vi "Intake Shooter Controller.vi"(8 "error in":errorcluster) -> ()   [LabVIEW 2019]
doc: "This VI executes continuously carrying out the current operation and responding to updates or new operations. It will often contain the timing or control code that is difficult to place directly in TeleOp. This VI generally opens all sensors and motors and isolates the rest of the robot code from knowing how the operations are carried out."
uses:
  <vilib>/Rock Robotics/WPI/Framework/Completion Status.ctl
  Intake Shooter Setpoints.ctl
  Intake Shooter Operations.ctl
  <vilib>/Rock Robotics/WPI/ThirdParty/REV Robotics/SPARK MAX/Typedef/Spark MAX Idle Mode.ctl
  <vilib>/Rock Robotics/WPI/ThirdParty/REV Robotics/SPARK MAX/Typedef/Spark MAX Control Type.ctl
  <vilib>/Rock Robotics/WPI/ThirdParty/Phoenix-LabVIEW/Motor Controller/Controls/CTRE_Phoenix_MotorControl_ControlMode.ctl
  <vilib>/Rock Robotics/Network Tables/NT Write Boolean.vi
panel:
  out "Iterations 3":i32
  out "Analog Position 2":dbl
  out "Iterations 2":i32
  out "Iterations":i32
  out "Analog Position":dbl
  in  "Interactive Values":T1
  out "Current\nCmd":string
  in  "Buttons":cluster{"Execute Cmd":bool, "Abort Cmd":bool}
  out "Command Timing":cluster{"Start Time (ms)":u32, "Iterations":i32}
  out "Status":T3
  # "Tip: It may be helpful to observe inputs and sensor values.\nYou may also want to display tuning or debugging controls."
  # "Interactive Command: You may fill in the settings for a command\nand schedule it with the Execute button. You can observe and abort\nany command while fine tuning the code for the controller."
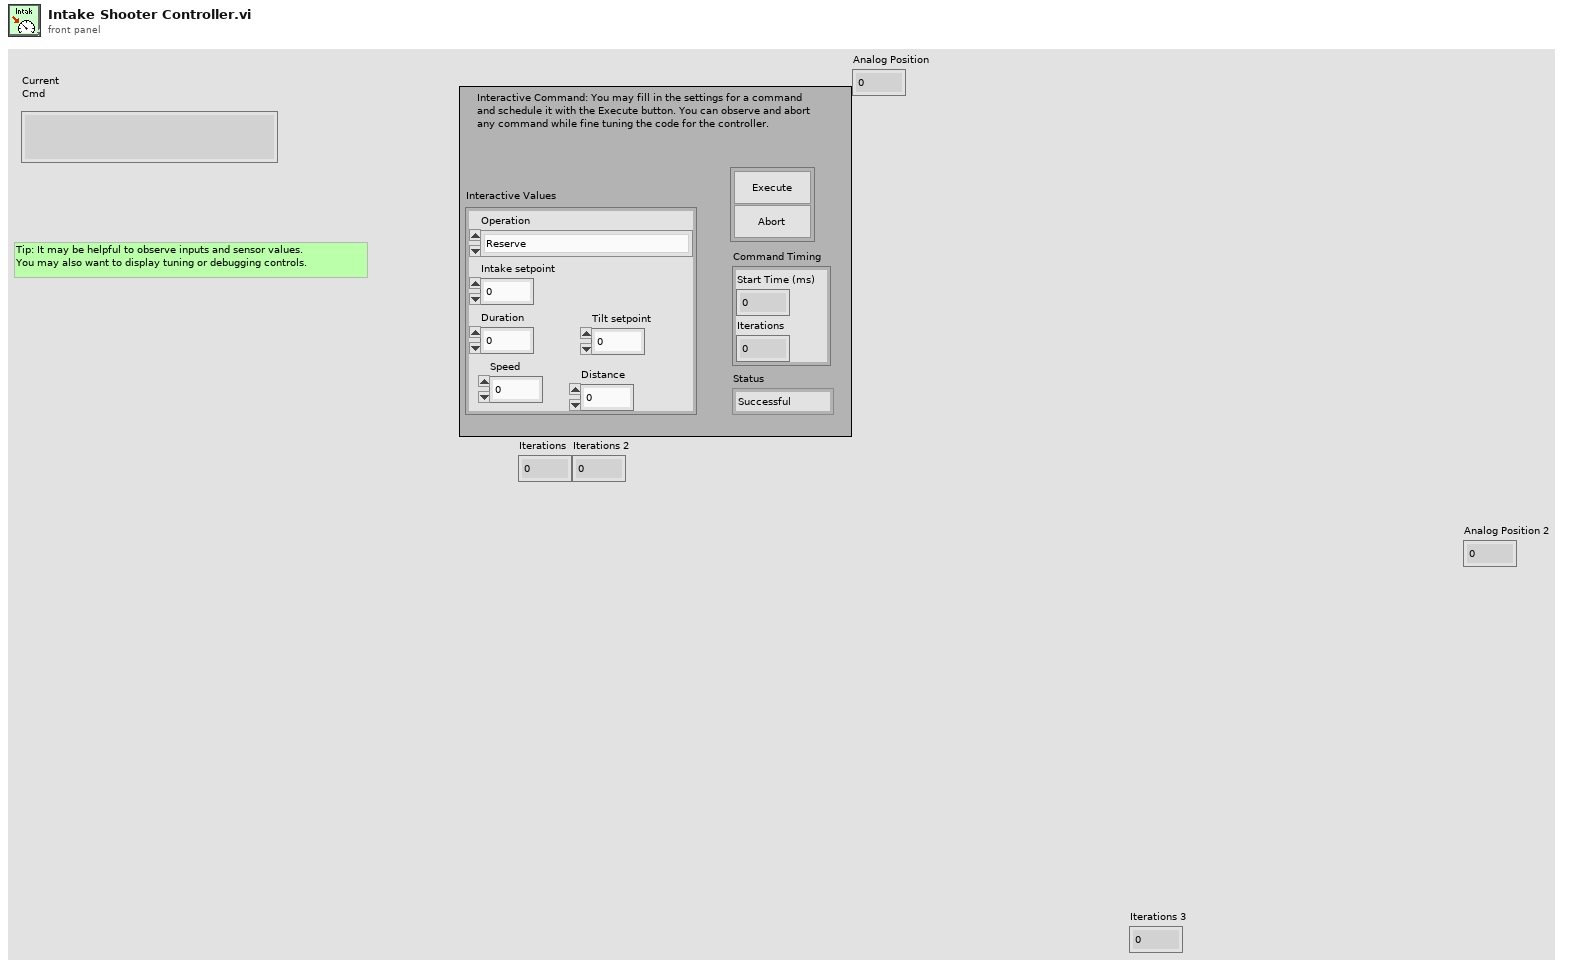
[diagram p1: front panel]
types:
  T1 = typedef "Intake Shooter Setpoints.ctl" = cluster{"Operation":T2, "Intake setpoint":dbl, "Duration":dbl, "Tilt setpoint":dbl, "Speed":dbl, "Distance":dbl}
  T2 = typedef "Intake Shooter Operations.ctl" = enum16{"Reserve", "Read Current", "Immediate", "Go up", "Go down", "Armediate"}
  T3 = typedef "Completion Status.ctl" = enum16{"Successful", "Aborted", "Incomplete"}
  T4 = typedef "Spark MAX Idle Mode.ctl" = enum16{"Coast", "Brake"}
  T5 = typedef "WPI_MotorControlDeviceRef.ctl" = cluster{"DeviceStatus":errorcluster, "Type":T6, "PWM":cluster{"PWM Channel":T7, "DeadBand":T8}, "CAN":cluster{"Device Number":u8, "SetOutput VI Ref":variant, "GetOutput VI Ref":variant, "Enable VI Ref":variant, "Disable VI Ref":variant, "Data":variant}, "Invert":bool, "DIO PWM":cluster{"PWM \"Enable\" Channel":T7, "DIOChannel":T9, "PWM Rate":dbl}}
  T6 = typedef "WPI_MotorControlType.ctl" = enum16{"PWM", "CAN", "DIO PWM"}
  T7 = typedef "FPGA_DIOPWMChannel.ctl" = enum8{"PWM 0", "PWM 1", "PWM 2", "PWM 3", "PWM 4", "PWM 5", "PWM 6", "PWM 7", "PWM 8", "PWM 9", "PWM MXP 0", "PWM MXP 1", "PWM MXP 2", "PWM MXP 3", "PWM MXP 4", "PWM MXP 5", "PWM MXP 6", "PWM MXP 7", "PWM MXP 8", "PWM MXP 9", "Invalid"}
  T8 = typedef "WPI_PWMDeadband.ctl" = cluster{"Name":string, "maxPositivePwm":i32, "minPositivePwm":i32, "centerPwm":i32, "maxNegativePwm":i32, "minNegativePwm":i32, "angularRange":u16}
  T9 = typedef "FPGA_DIOChannel.ctl" = enum8{"DIO 0", "DIO 1", "DIO 2", "DIO 3", "DIO 4", "DIO 5", "DIO 6", "DIO 7", "DIO 8", "DIO 9", "DIO MXP 0", "DIO MXP 1", "DIO MXP 2", "DIO MXP 3", "DIO MXP 4", "DIO MXP 5", "DIO MXP 6", "DIO MXP 7", "DIO MXP 8", "DIO MXP 9", "DIO MXP 10", "DIO MXP 11", "DIO MXP 12", "DIO MXP 13", "DIO MXP 14", "DIO MXP 15", "SPI Port CS1", "SPI Port CS2", "SPI Port CS3", "SPI Port MISO", "SPI Port MOSI", "Invalid"}
  T10 = typedef "Command Status Info.ctl" = cluster{"Name":string, "Status":T3, "notifier out":T11}
  T11 = typedef "Completion Notifier.ctl" = refnum<notifier>
  T12 = cluster{"Current Command":T1, "Command Timing":cluster{"Start Time (ms)":u32, "Iterations":i32}, "Command Arguments":cluster{"Command Info":T10, "Description":string, "Default Command":T1, "queue out":refnum<queue>, "Subsystem Name":string}}
  T13 = typedef "Spark MAX Control Type.ctl" = enum16{"Percent VBus", "Voltage", "Velocity", "Position", "Smart Motion", "Current", "Smart Velocity"}
  T14 = typedef "CTRE_Phoenix_MotorControl_ControlMode.ctl" = u16
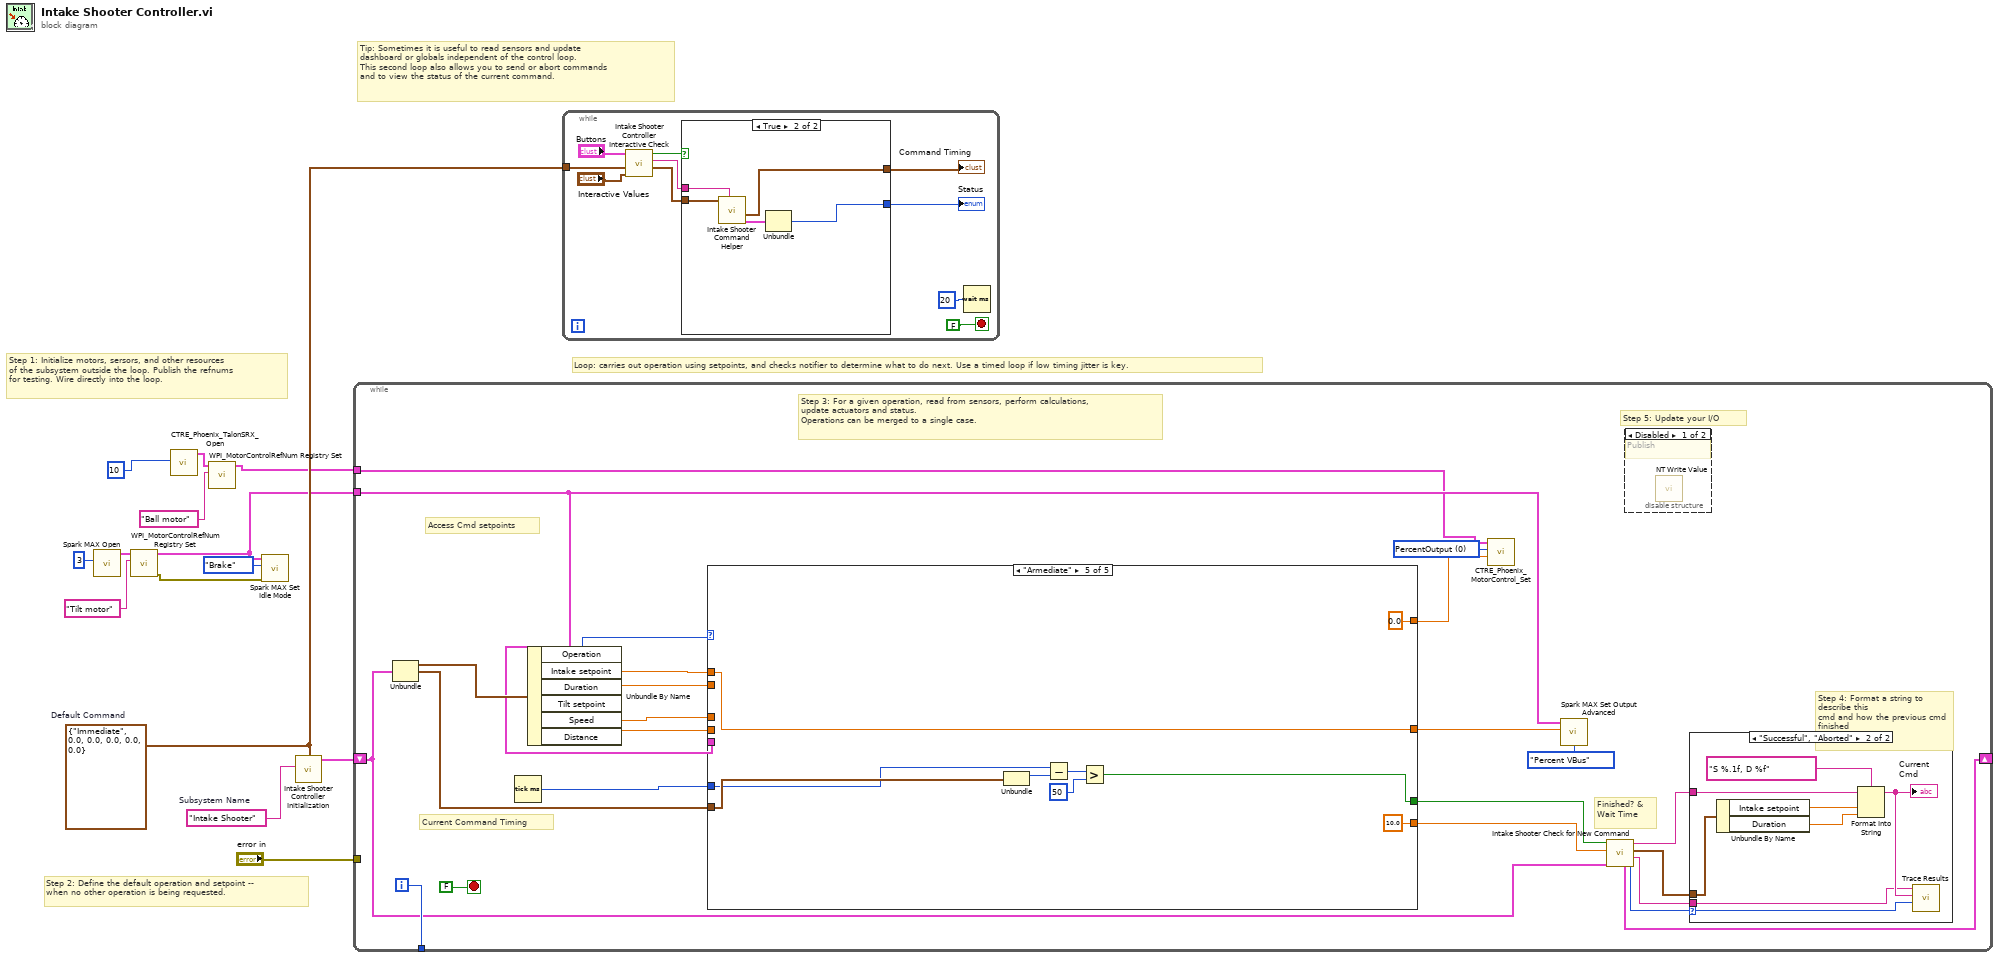
[diagram p0: block diagram]
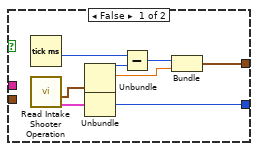
[diagram p2: hidden frame]
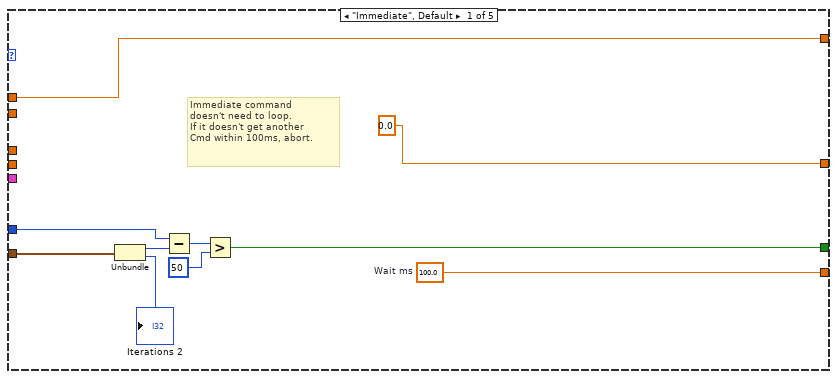
[diagram p4: hidden frame]
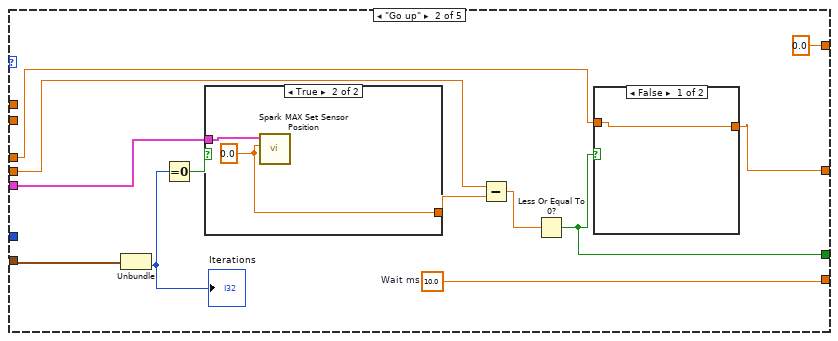
[diagram p5: hidden frame]
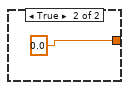
[diagram p6: hidden frame]
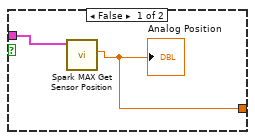
[diagram p7: hidden frame]
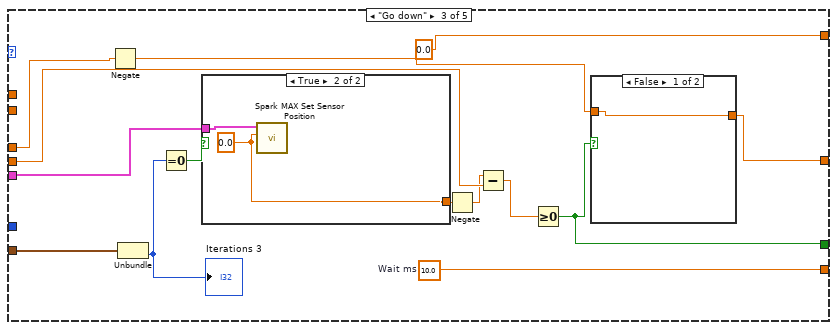
[diagram p8: hidden frame]
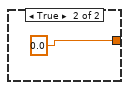
[diagram p9: hidden frame]
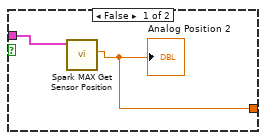
[diagram p10: hidden frame]
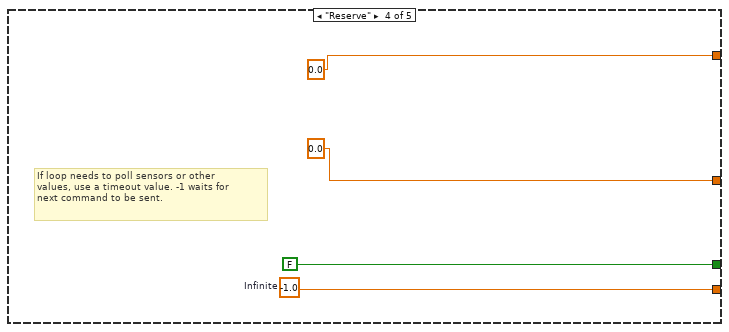
[diagram p11: hidden frame]
diagram:
  w11 = T1 {"Operation"=enum."Immediate", "Intake setpoint"=0.0, "Duration"=0.0, "Tilt setpoint"=0.0, "Speed"=0.0, "Distance"=0.0}  # Default Command
  w12 = "Intake Shooter"  # Subsystem Name
  # "Tip: Sometimes it is useful to read sensors and update\ndashboard or globals independent of the control loop.\nThis second loop also allows you to send or abort commands\nand to view the status of the current command."
  # "Step 2: Define the default operation and setpoint --\nwhen no other operation is being requested."
  # "Step 1: Initialize motors, sersors, and other resources\nof the subsystem outside the loop. Publish the refnums\nfor testing. Wire directly into the loop."
  # "Loop: carries out operation using setpoints, and checks notifier to determine what to do next. Use a timed loop if low timing jitter is key."
  n1 = call <vilib>:"Spark MAX Open.vi"("Device Number"=u8 3) -> ("MotorControlDeviceRef"=w9:T5)  [unwired: 9 in, 1 out]
  n2 = call <vilib>:"WPI_MotorControlRefNum Registry Set.vi"("refnum name"="Tilt motor", "MotorControlDevRef"=w9) -> ("error out"=w3:errorcluster, "MotorControlDevRef"=w2:T5)  [unwired: 8 in]
  n3 = call <vilib>:"CTRE_Phoenix_TalonSRX_Open.vi"("Device Number"=u8 10) -> ("CAN Talon SRX Ref"=w4:T5)  [unwired: 9 in, 1 out]
  n4 = call <vilib>:"WPI_MotorControlRefNum Registry Set.vi"("refnum name"="Ball motor", "MotorControlDevRef"=w4) -> ("MotorControlDevRef"=w6:T5)  [unwired: 8 in, 1 out]
  n5 = call <vilib>:"Spark MAX Set Idle Mode.vi"("error in (no error)"=w3, "Idle Mode"=Spark_MAX_Idle_Mode."Brake", "MotorControlDeviceRef in"=w2) -> ()  [unwired: 7 in, 2 out]
  n6 = call "Intake Shooter Controller Initialization.vi"("Subsystem Name"=w12, "Default Command"=w11) -> ("Current Command"=w13:T12)  [unwired: 9 in]
  n7 = while {
    shift-right: [w31] -> _
    shift-left: w13 -> [w24]
    tunnel: [w37] -> _
    tunnel: "error in" -> [_]
    tunnel: w6 -> [w17]
    tunnel: w2 -> [w19]
    i -> [w37]
    stop <- FALSE stop-if-true
    w15 = T14 0 items=["PercentOutput"=0, "Position"=1, "Velocity"=2, "Current"=3, "Follower"=5, "MotionProfile"=6, "MotionMagic"=7, "MotionProfileArc"=10, "Disabled"=15] ("Control Mode")
    # "Step 5: Update your I/O"
    # "Step 4: Format a string to describe this\ncmd and how the previous cmd finished"
    # "Current Command Timing"
    # "Access Cmd setpoints"
    # "Finished? &\nWait Time"
    # "Step 3: For a given operation, read from sensors, perform calculations,\nupdate actuators and status.\nOperations can be merged to a single case."
    n8 = Unbundle(w24) -> ("Current Command"=w36:T1, "Command Timing"=w33:cluster{"Start Time (ms)":u32, "Iterations":i32})  [unwired: 1 out]
    n9 = Tick Count (ms)() -> (millisecond timer value=w34:u32)
    n10 = Unbundle By Name(w36) -> ("Operation"=w35:T2, "Intake setpoint"=w32:dbl, "Duration"=w22:dbl, "Speed"=w21:dbl, "Distance"=w20:dbl)  [unwired: 1 out]
    n11 = case shown="\"Armediate\"" w35 {
      tunnel: [w48 w60 w71 w90 10.0 ("Infinite")] -> w29
      tunnel: [w42 w50 w72 FALSE ("ignore previous (F)") w93] -> w30
      tunnel: w33 -> [w44 w59 w70 _ w94]
      tunnel: w34 -> [w43 _ _ _ w92]
      tunnel: w32 -> [w41 _ _ _ w98]
      tunnel: [w41 0.0 ("f") 0.0 ("f") 0.0 ("f") 0.0 ("f")] -> w16
      tunnel: [0.0 ("Setpoint") w52 w73 0.0 w98] -> w23
      tunnel: w19 -> [_ w56 w76 _ _]
      tunnel: w22 -> [_ _ _ _ _]
      tunnel: w21 -> [_ w51 w75 _ _]
      tunnel: w20 -> [_ w55 w69 _ _]
      frame "Immediate", Default {
        w48 = 100.0  # Wait ms
        # "Immediate command\ndoesn't need to loop.\nIf it doesn't get another\nCmd within 100ms, abort."
        n12 = Unbundle(w44) -> ("Start Time (ms)"=w47:u32, "Iterations"=→"Iterations 2":i32)
        n13 = Subtract(x=w43, y=w47) -> (x-y=w46:u32)
        n14 = Greater?(x=w46, y=u8 50 ("Left Motor")) -> (0:w42:bool)
      }
      frame "Go up" {
        w60 = 10.0  # Wait ms
        n15 = Unbundle(w59) -> ("Iterations"=w58:i32)  [unwired: 1 out]
        "Iterations" <- w58
        n16 = Equal To 0?(x=w58) -> (x = 0?=w57:bool)
        n17 = case shown="True" w57 {
          tunnel: w56 -> [w63 w66]
          tunnel: [w64 w65] -> w54
          frame False {
            n18 = call <vilib>:"Spark MAX Get Sensor Position.vi"("MotorControlDevRef in"=w63) -> ("Sensor Position"=w64:dbl)  [unwired: 7 in, 3 out]
            "Analog Position" <- w64
          }
          frame True {
            w65 = 0.0 ("Position")
            n19 = call <vilib>:"Spark MAX Set Sensor Position.vi"("Position"=w65, "MotorControlDeviceRef"=w66) -> ()  [unwired: 8 in, 2 out]
          }
        }
        n20 = Subtract(x=w55, y=w54) -> (x-y=w53:dbl)
        n21 = Less Or Equal To 0?(x=w53) -> (x <= 0?=w50:bool)
        n22 = case shown="False" w50 {
          tunnel: [w61 0.0 ("Setpoint")] -> w52
          tunnel: w51 -> [w61 _]
          frame False {
          }
          frame True {
          }
        }
      }
      frame "Go down" {
        w71 = 10.0  # Wait ms
        n23 = Negate(x=w75) -> (-x=w74:dbl)
        n24 = Unbundle(w70) -> ("Iterations"=w79:i32)  [unwired: 1 out]
        "Iterations 3" <- w79
        n25 = Equal To 0?(x=w79) -> (x = 0?=w78:bool)
        n26 = case shown="True" w78 {
          tunnel: w76 -> [w83 w86]
          tunnel: [w84 w85] -> w68
          frame False {
            n27 = call <vilib>:"Spark MAX Get Sensor Position.vi"("MotorControlDevRef in"=w83) -> ("Sensor Position"=w84:dbl)  [unwired: 7 in, 3 out]
            "Analog Position 2" <- w84
          }
          frame True {
            w85 = 0.0 ("Position")
            n28 = call <vilib>:"Spark MAX Set Sensor Position.vi"("Position"=w85, "MotorControlDeviceRef"=w86) -> ()  [unwired: 8 in, 2 out]
          }
        }
        n29 = Negate(x=w68) -> (-x=w67:dbl)
        n30 = Subtract(x=w67, y=w69) -> (x-y=w77:dbl)
        n31 = Greater Or Equal To 0?(x=w77) -> (x >= 0?=w72:bool)
        n32 = case shown="False" w72 {
          tunnel: [w81 0.0 ("Setpoint")] -> w73
          tunnel: w74 -> [w81 _]
          frame False {
          }
          frame True {
          }
        }
      }
      frame "Reserve" {
        w90 = -1.0  # Infinite
        # "If loop needs to poll sensors or other\nvalues, use a timeout value. -1 waits for\nnext command to be sent."
      }
      frame "Armediate" {
        n33 = Unbundle(w94) -> ("Start Time (ms)"=w96:u32)  [unwired: 1 out]
        n34 = Subtract(x=w92, y=w96) -> (x-y=w97:u32)
        n35 = Greater?(x=w97, y=u8 50 ("Left Motor")) -> (0:w93:bool)
      }
    }
    n36 = call <vilib>:"CTRE_Phoenix_MotorControl_Set.vi"("Output"=w16, "Control Mode"=w15, "PhoenixMotorControlDevRef"=w17) -> ()  [unwired: 7 in, 2 out]
    n37 = call <vilib>:"Spark MAX Set Output Advanced.vi"("Control Mode"=Spark_MAX_Control_Type."Percent VBus", "Setpoint"=w23, "MotorControlDevRef"=w19) -> ()  [unwired: 7 in, 2 out]
    n38 = call "Intake Shooter Check for New Command.vi"("Current Command"=w24, "Wait time (ms)"=w29, "Finished?"=w30) -> ("Completion"=w25:T3, "Subsystem Name"=w26:string, "Current Command"=w27:T1, "Initial Trace String"=w28:string, "NextCommand"=w31:T12)  [unwired: 4 in]
    n39 = disable-structure shown="Disabled" {
      frame Disabled {
        # "Publish"
        n40 = call-poly <vilib>:"NT Write Value.vi"() -> ()  [unwired: 11 in, 1 out]
      }
      frame Enabled {
      }
    }
    n41 = case shown="\"Successful\", \"Aborted\"" w25 {
      selector: w25 -> [_ w107]
      tunnel: w28 -> [_ w103]
      tunnel: w27 -> [_ w104]
      tunnel: w26 -> [_ w100]
      frame "Incomplete", Default {
        # "Continuing current command"
      }
      frame "Successful", "Aborted" {
        # "Report and setup for next command"
        n42 = Unbundle By Name(w104) -> ("Intake setpoint"=w106:dbl, "Duration"=w101:dbl)
        n43 = Format Into String(format string="S %.1f, D %f", initial string=w103, w106, w101) -> (resulting string=w102:string)  [unwired: 1 in, 1 out]
        "Current\nCmd" <- w102
        n44 = call <vilib>:"Trace Results.vi"("Status of previous command"=w107, "Description"=w102, "Subsystem"=w100) -> ()  [unwired: 9 in]
      }
    }
  }
  n45 = while {
    tunnel: w11 -> [w114]
    stop <- FALSE stop-if-true
    n46 = call "Intake Shooter Controller Interactive Check.vi"("Interactive Command in"="Interactive Values", "Default Command"=w114, "Buttons"="Buttons") -> ("Interactive Command out"=w111:T1, "Trace String"=w112:string, "Schedule"=w113:bool)  [unwired: 6 in]
    n47 = case shown="True" w113 {
      tunnel: [w125 w130] -> w110
      tunnel: w111 -> [_ w128]
      tunnel: [w121 w126] -> w109
      tunnel: w112 -> [_ w129]
      frame False {
        n48 = Tick Count (ms)() -> (millisecond timer value=w120:u32)
        n49 = call "Read Intake Shooter Operation.vi"() -> ("Command Info"=w118:T10, "SubSystem Data"=w119:T1)  [unwired: 9 in, 1 out]
        n50 = Unbundle(w119) -> ("Operation"=w124:T2, "Intake setpoint"=w122:dbl)  [unwired: 4 out]
        n51 = Unbundle(w118) -> ("Status"=w125:T3)  [unwired: 2 out]
        n52 = Subtract(x=w120, y=w124) -> (x-y=w123:u32)
        n53 = Bundle(w123, "Intake setpoint"=w122) -> (w121:cluster{u32, "Intake setpoint":dbl})  [unwired: 1 in]
      }
      frame True {
        n54 = call "Intake Shooter Command Helper.vi"("Description"=w129, "SubSystem Data"=w128) -> ("Command Info Out"=w127:T10, "Command Timing"=w126:cluster{"Start Time (ms)":u32, "Iterations":i32})  [unwired: 7 in, 1 out]
        n55 = Unbundle(w127) -> ("Status"=w130:T3)  [unwired: 2 out]
      }
    }
    "Status" <- w110
    "Command Timing" <- w109
    n56 = Wait (ms)(milliseconds to wait=u32 20) -> ()  [unwired: 1 out]
  }
